vi "UploadToTarget.vi"(8 "error in (no error)":errorcluster, 9 "previousName":string, 10 "ConnectionData":T3, 11 "ConfigXMLControls":T1) -> (0 "error out":errorcluster, 3 "newName":string)   [LabVIEW 2016]
uses:
  General/RemoteFiles/connectionData.ctl
  ConfigXMLControl.ctl
  General/CorePluginInfo.ctl
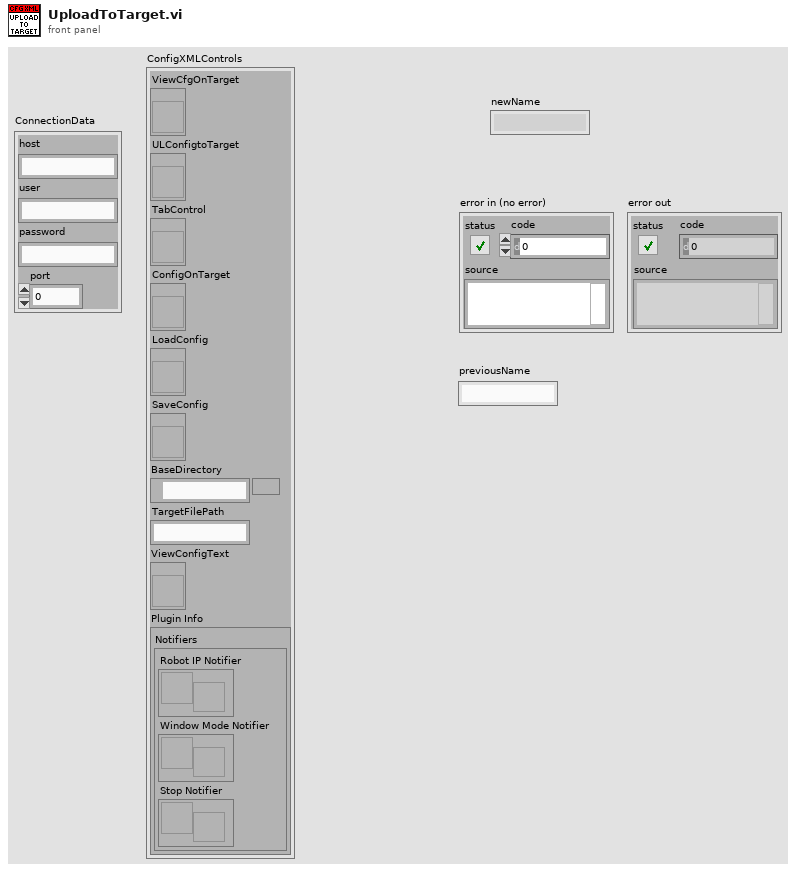
[diagram p1: front panel]
types:
  T1 = typedef "ConfigXMLControl.ctl" = cluster{"ViewCfgOnTarget":refnum<vi>, "ULConfigtoTarget":refnum<vi>, "TabControl":refnum<vi>, "ConfigOnTarget":refnum<vi>, "LoadConfig":refnum<vi>, "SaveConfig":refnum<vi>, "BaseDirectory":path, "TargetFilePath":string, "ViewConfigText":refnum<vi>, "Plugin Info":T2}
  T2 = typedef "CorePluginInfo.ctl" = cluster{"Notifiers":cluster{"Robot IP Notifier":refnum<notifier>, "Window Mode Notifier":refnum<notifier>, "Stop Notifier":refnum<notifier>}}
  T3 = typedef "connectionData.ctl" = cluster{"host":string, "user":string, "password":string, "port":u16}
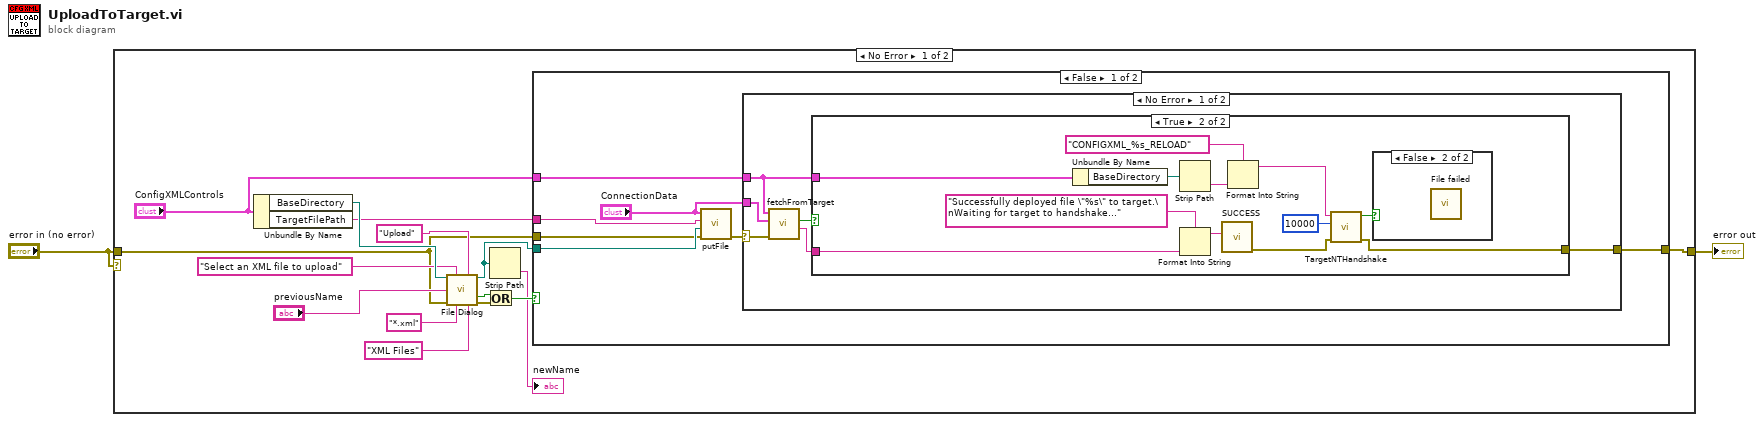
[diagram p0: block diagram]
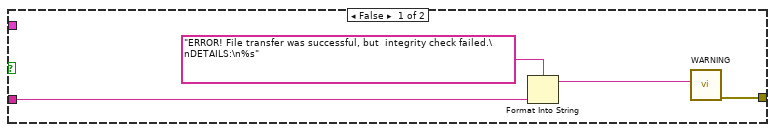
[diagram p2: hidden frame]
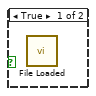
[diagram p3: hidden frame]
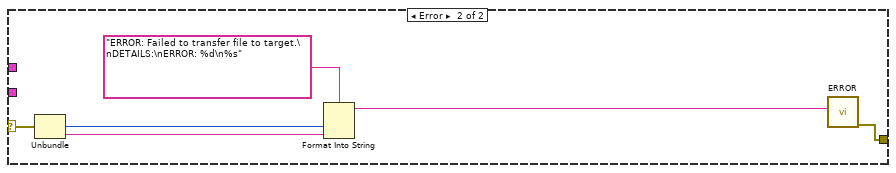
[diagram p4: hidden frame]
diagram:
  n1 = case shown="No Error" "error in (no error)" {
    tunnel: "error in (no error)" -> [w7 w54]
    tunnel: [w5 w54] -> w1
    frame No Error {
      n2 = Unbundle By Name("ConfigXMLControls") -> ("BaseDirectory"=w14:path, "TargetFilePath"=w8:string)
      n3 = call "File Dialog"("start path"=w14, "prompt"="Select an XML file to upload", "button label"="Upload", "default name"="previousName", "error in"=w7, "pattern (all files)"="*.xml", "pattern label"="XML Files") -> ("selected path"=w4:path, "cancelled"=w11:bool, "error out"=w10:errorcluster)  [unwired: 5 in, 1 out]
      n4 = Or(x=w11, y=w10) -> (x .or. y?=w9:bool)
      n5 = Strip Path(path=w4) -> (name=→"newName":string)  [unwired: 1 out]
      n6 = case shown="False" w9 {
        tunnel: w4 -> [w23 _]
        tunnel: w8 -> [w24 _]
        tunnel: w7 -> [w22 w53]
        tunnel: "ConfigXMLControls" -> [w19 _]
        tunnel: [w18 w53] -> w5
        frame False {
          n7 = call "putFile.vi"("error in (no error)"=w22, "local path"=w23, "remote path"=w24, "ConnectionData"="ConnectionData") -> ("error out"=w21:errorcluster)  [unwired: 6 in, 1 out]
          n8 = case shown="No Error" w21 {
            selector: w21 -> [w29 w51]
            tunnel: "ConnectionData" -> [w30 _]
            tunnel: w19 -> [w25 _]
            tunnel: [w26 w47] -> w18
            frame No Error {
              n9 = call "fetchFromTarget.vi"("error in (no error)"=w29, "ConnectionData"=w30, "ConfigXMLControls"=w25) -> ("nameMessageOut"=w27:string, "SuccessfulRead?"=w28:bool)  [unwired: 4 in, 3 out]
              n10 = case shown="True" w28 {
                tunnel: w27 -> [w33 w45]
                tunnel: [w31 w35] -> w26
                tunnel: w25 -> [_ w43]
                frame False {
                  n11 = Format Into String(format string="ERROR! File transfer was successful, but  integrity check failed.\nDETAILS:\n%s" ("Message"), w33) -> (resulting string=w32:string)  [unwired: 2 in, 1 out]
                  n12 = call "WARNING"("Message"=w32) -> ("error out"=w31:errorcluster)  [unwired: 9 in, 1 out]
                }
                frame True {
                  n13 = Unbundle By Name(w43) -> ("BaseDirectory"=w42:path)
                  n14 = Strip Path(path=w42) -> (name=w40:string)  [unwired: 1 out]
                  n15 = Format Into String(format string="Successfully deployed file \"%s\" to target.\nWaiting for target to handshake..." ("Message"), w45) -> (resulting string=w44:string)  [unwired: 2 in, 1 out]
                  n16 = call "SUCCESS"("Message"=w44) -> ("error out"=w36:errorcluster)  [unwired: 9 in, 1 out]
                  n17 = Format Into String(format string="CONFIGXML_%s_RELOAD", w40) -> (resulting string=w39:string)  [unwired: 2 in, 1 out]
                  n18 = call "TargetNTHandshake.vi"("error in"=w36, "Timeout"=10000, "Name"=w39) -> ("error out"=w35:errorcluster, "Acknowledged"=w37:bool)  [unwired: 7 in]
                  n19 = case shown="False" w37 {
                    frame True {
                      n20 = call "File Loaded"() -> ()  [unwired: 10 in, 2 out]
                    }
                    frame False {
                      n21 = call "File failed"() -> ()  [unwired: 10 in, 2 out]
                    }
                  }
                }
              }
            }
            frame Error {
              n22 = Unbundle(w51) -> ("code"=w50:i32, "source"=w49:string)  [unwired: 1 out]
              n23 = Format Into String(format string="ERROR: Failed to transfer file to target.\nDETAILS:\nERROR: %d\n%s", w50, w49) -> (resulting string=w48:string)  [unwired: 2 in, 1 out]
              n24 = call "ERROR"("Message"=w48) -> ("error out"=w47:errorcluster)  [unwired: 9 in, 1 out]
            }
          }
        }
        frame True {
          # "If true, do not upload"
        }
      }
    }
    frame Error {
    }
  }
  "error out" <- w1
